vi "DHE_set_roi.vi"(0 "fd":i32, 1 "xlenght":i32, 2 "ylenght":i32, 5 "xstart":i32, 7 "ystart":i32, 11 "error in (no error)":errorcluster) -> (4 "fd out":i32, 8 "return value":i32, 15 "error out":errorcluster)   [LabVIEW 2016]
doc: "This VI closes the I/O interface with the instrument."
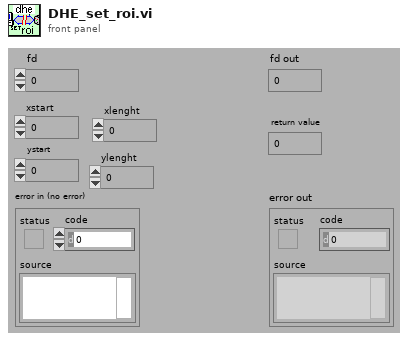
[diagram p1: front panel]
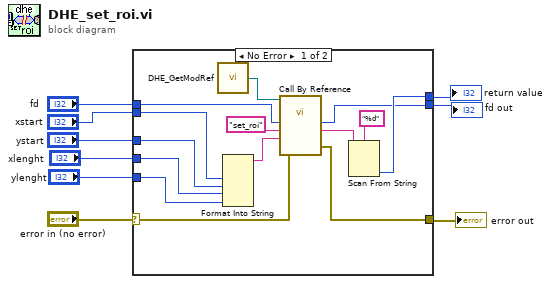
[diagram p0: block diagram]
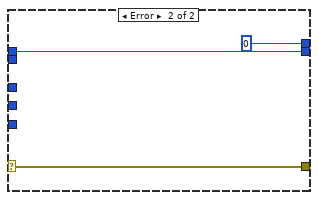
[diagram p2: hidden frame]
diagram:
  n1 = case shown="No Error" "error in (no error)" {
    selector: "error in (no error)" -> [w18 w24]
    tunnel: "fd" -> [w14 w26]
    tunnel: [w16 0] -> w8
    tunnel: [w17 w24] -> w7
    tunnel: "xstart" -> [w13 _]
    tunnel: "ystart" -> [w12 _]
    tunnel: [w15 w26] -> w4
    tunnel: "xlenght" -> [w11 _]
    tunnel: "ylenght" -> [w10 _]
    frame No Error {
      n2 = call "DHE_GetModRef.vi"() -> ("DHE_ModRef"=w23:refnum<vi>)  [unwired: 9 out]
      n3 = Format Into String(w13, w12, w11, w10) -> (resulting string=w19:string)  [unwired: 3 in, 1 out]
      n4 = call-by-ref "?"(reference=w23, "error in (no error)"=w18, "arguments"=w19, "function"="set_roi", "fd in"=w14) -> ("error out"=w17:errorcluster, "str result"=w21:string, "fd out"=w15:i32)  [unwired: 5 in, 3 out]
      n5 = Scan From String(format string="%d", input string=w21) -> (output 1=w16:i32)  [unwired: 2 in, 4 out]
    }
    frame Error {
    }
  }
  "error out" <- w7
  "return value" <- w8
  "fd out" <- w4
